vi "Host.vi"() -> ()   [LabVIEW 2025]
uses:
  Controls/panel select 2.ctl
  Controls/home button.ctl
  Controls/manual button 2.ctl
  Controls/edit programs button.ctl
  Controls/diagnostics button.ctl
  Controls/info button 2.ctl
  <vilib>/Handler Framework/CmdQueue/Enqueue Single.vi
  <vilib>/Handler Framework/Handler Framework.lvlib
panel:
  out "Modules":T1
  in  "Page Select":T2
  # "Energized Bake Oven"
  # "Version 1.0.0.0"
  # "RAM Aerospace\nSt. George, UT, 84790\nLabVIEW 2025 Q1\nDQMH-LVOOP-HAL"
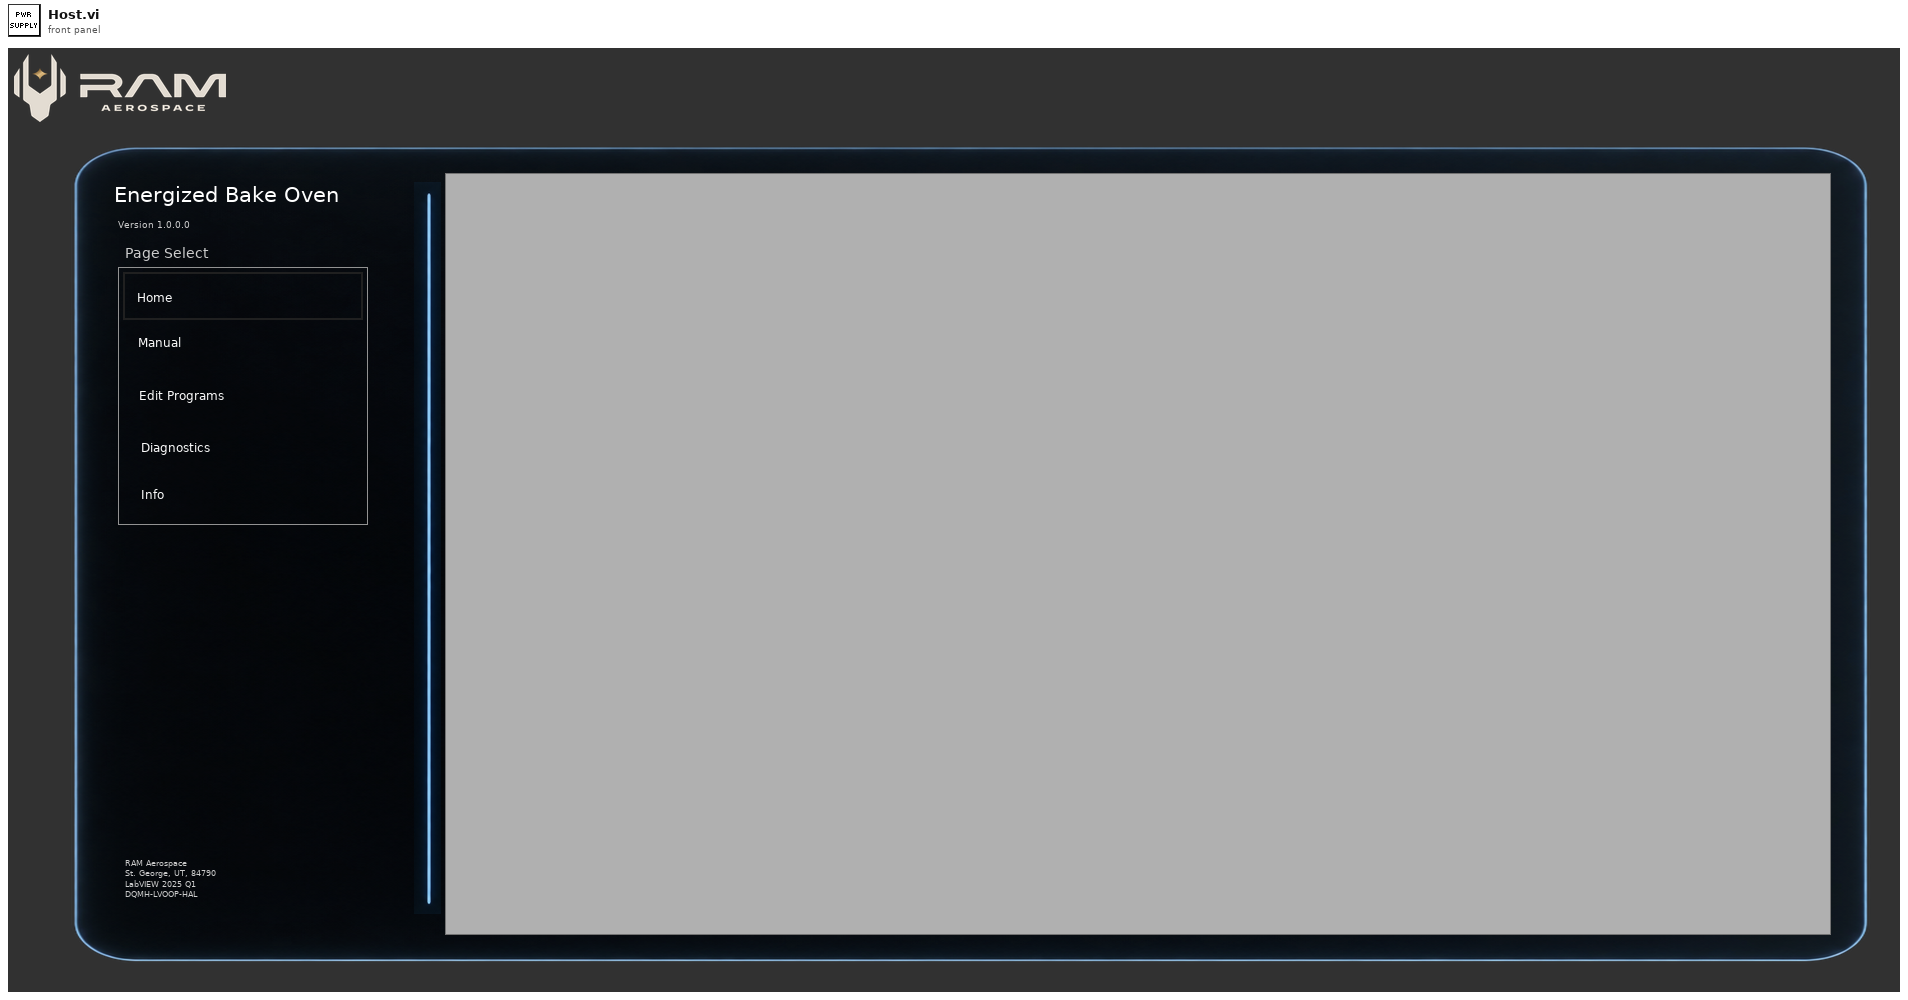
[diagram p1: front panel]
types:
  T1 = cluster{"Module IDs":i32[], "Module Names":string[]}
  T2 = typedef "panel select 2.ctl" = enum32{"Home", "Manual", "Edit Programs", "Diagnostics", "Info"}
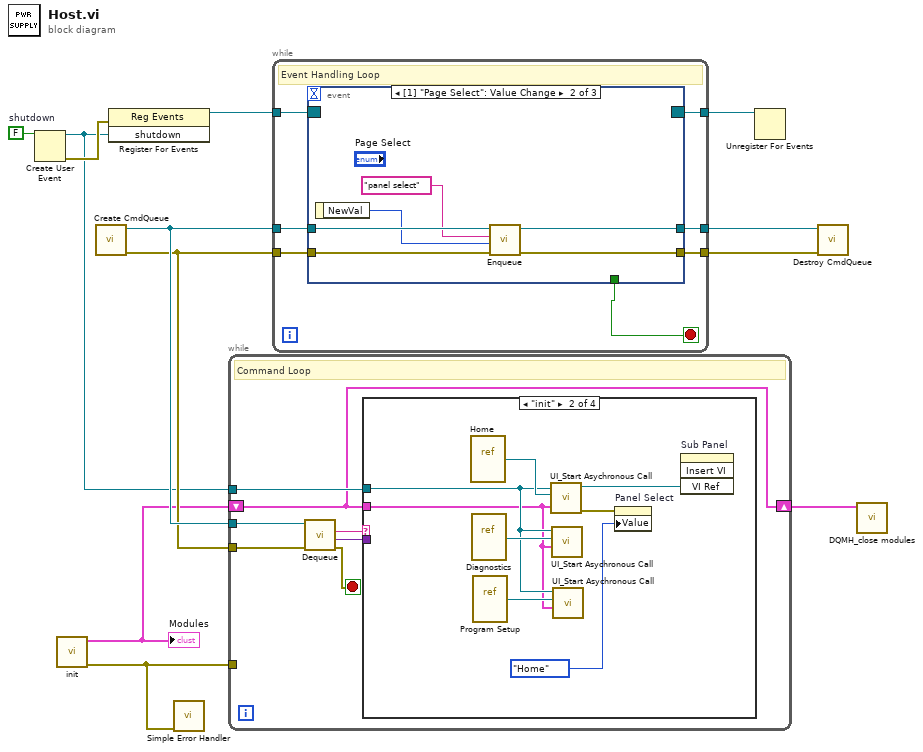
[diagram p0: block diagram]
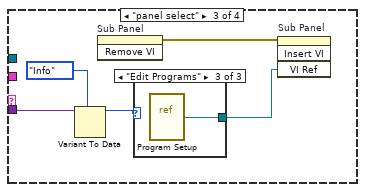
[diagram p3: hidden frame]
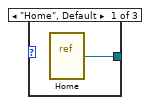
[diagram p4: hidden frame]
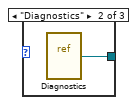
[diagram p5: hidden frame]
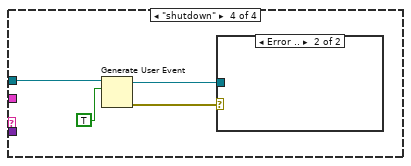
[diagram p6: hidden frame]
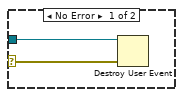
[diagram p7: hidden frame]
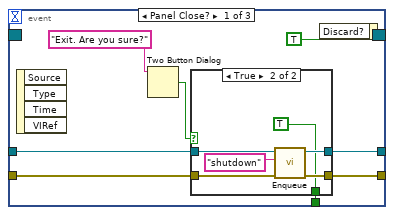
[diagram p8: hidden frame]
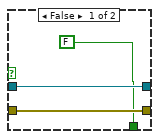
[diagram p9: hidden frame]
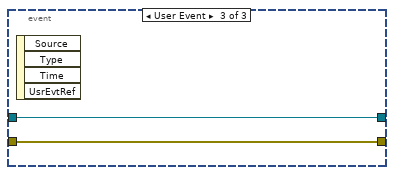
[diagram p10: hidden frame]
diagram:
  w8 = FALSE  # shutdown
  n1 = Create User Event(user event datatype=w8) -> (user event=w4:refnum<user-event>, error out=w5:errorcluster)  [unwired: 1 in]
  n2 = call "init.vi"() -> ("error out"=w1:errorcluster, "Modules"=w3:T1)  [unwired: 10 in]
  "Modules" <- w3
  n3 = call <vilib>:"Create CmdQueue.vi"() -> ("error out"=w9:errorcluster, "CmdQueue out"=w10:refnum<queue>)  [unwired: 10 in]
  n4 = register-events(error in=w5, w4) -> (reference out=w7:refnum<event-registration>)  [unwired: 1 in, 1 out]
  n5 = call <vilib>:"Simple Error Handler.vi"("error in (no error)"=w1) -> ()  [unwired: 4 in, 5 out]
  n6 = while {
    tunnel: w10 -> [w19]
    tunnel: w9 -> [w16]
    tunnel: w4 -> [w15]
    tunnel: w1 -> [_]
    shift-right: [w13] -> w2
    shift-left: w3 -> [w13]
    stop <- w14 stop-if-true
    # "Command Loop"
    n7 = call <vilib>:"Dequeue.vi"("error in (no error)"=w16, "CmdQueue in"=w19) -> ("error out"=w14:errorcluster, "value"=w17:variant, "cmd"=w18:string)  [unwired: 5 in, 2 out]
    n8 = case shown="\"init\"" w18 {
      tunnel: w17 -> [_ _ w32 _]
      tunnel: w15 -> [_ w23 _ w39]
      tunnel: w13 -> [_ w22 _ _]
      frame "False", Default {
      }
      frame "init" {
        n9 = vi-ref "Home.vi"() -> (w27:refnum<vi>)
        n10 = vi-ref "Diagnostics.vi"() -> (w26:refnum<vi>)
        n11 = vi-ref "Program Setup.vi"() -> (w24:refnum<vi>)
        n12 = call "UI_Start Asychronous Call.vi"("DQMH Modules"=w22, "VI Refnum"=w27, "User Event in"=w23) -> ("error out"=w21:errorcluster, "VI ref"=w25:refnum<vi>)  [unwired: 7 in]
        n13 = call "UI_Start Asychronous Call.vi"("DQMH Modules"=w22, "VI Refnum"=w26, "User Event in"=w23) -> ()  [unwired: 7 in, 2 out]
        n14 = call "UI_Start Asychronous Call.vi"("DQMH Modules"=w22, "VI Refnum"=w24, "User Event in"=w23) -> ()  [unwired: 7 in, 2 out]
        n15 = property on="Panel Select" class="RadioBtnsControl (strict)"(error in=w21, "Value"=panel_select_2."Home" ("Panel Select")) -> ()  [unwired: 1 in, 2 out]
        n16 = invoke on="Sub Panel" class="SubPnl" method="Insert VI"("VI Ref"=w25) -> ()  [unwired: 3 in, 4 out]
      }
      frame "panel select" {
        n17 = Variant To Data(type=panel_select_2."Info" ("Panel Select"), Variant=w32) -> (data=w31:T2)  [unwired: 1 in, 1 out]
        n18 = invoke on="Sub Panel" class="SubPnl" method="Remove VI"() -> (error out=w30:errorcluster)  [unwired: 3 in, 2 out]
        n19 = case shown="\"Edit Programs\"" w31 {
          tunnel: [w33 w34 w35] -> w29
          frame "Home", Default {
            n20 = vi-ref "Home.vi"() -> (w33:refnum<vi>)
          }
          frame "Diagnostics" {
            n21 = vi-ref "Diagnostics.vi"() -> (w34:refnum<vi>)
          }
          frame "Edit Programs" {
            n22 = vi-ref "Program Setup.vi"() -> (w35:refnum<vi>)
          }
        }
        n23 = invoke on="Sub Panel" class="SubPnl" method="Insert VI"(error in=w30, "VI Ref"=w29) -> ()  [unwired: 2 in, 4 out]
      }
      frame "shutdown" {
        n24 = Generate User Event(user event=w39, event data cluster=TRUE ("event data")) -> (user event out=w37:refnum<user-event>, error out=w36:errorcluster)  [unwired: 2 in]
        n25 = case shown="Error .." w36 {
          selector: w36 -> [w40 _]
          tunnel: w37 -> [w41 _]
          frame No Error {
            n26 = Destroy User Event(user event=w41, error in=w40) -> ()  [unwired: 1 out]
          }
          frame Error {
          }
        }
      }
    }
  }
  n27 = while {
    tunnel: w10 -> [w46]
    tunnel: [w44] -> w12
    tunnel: w9 -> [w45]
    tunnel: [w43] -> w11
    tunnel: w7 -> [w48]
    tunnel: [w47] -> w6
    stop <- w42 stop-if-true
    # "Event Handling Loop"
    n28 = event shown="[1] \"Page Select\": Value Change" {
      selector: w48 -> [_ _ _]
      dyn-events: [_ _ _] -> w47
      timeout: _ -> [_ _ _]
      tunnel: w46 -> [w56 w71 w73]
      tunnel: w45 -> [w55 w68 w72]
      tunnel: [w53 w70 w73] -> w44
      tunnel: [w52 w69 w72] -> w43
      tunnel: [w49 _ _] -> w42
      event Panel Close? {
        n29 = event-data() -> ()  [unwired: 1 in, 4 out]
        n30 = Two Button Dialog(message="Exit. Are you sure?") -> (T button?=w50:bool)  [unwired: 2 in]
        n31 = case shown="True" w50 {
          tunnel: w56 -> [w59 w64]
          tunnel: w55 -> [w58 w63]
          tunnel: [w59 w62] -> w53
          tunnel: [w58 w61] -> w52
          tunnel: [FALSE ("T button?") TRUE ("T button?")] -> w49
          frame False {
          }
          frame True {
            n32 = call-poly <vilib>:"Enqueue.vi"("error in (no error)"=w63, "Command"="shutdown", "CmdQueue in"=w64) -> ("error out"=w61:errorcluster, "CmdQueue out"=w62:refnum<queue>)  [unwired: 7 in]
          }
        }
        n33 = event-data("Discard?"=TRUE) -> ()  [unwired: 1 in, 1 out]
      }
      event Value Change {
        n34 = event-data() -> ("NewVal"=w66:T2)  [unwired: 1 in]
        n35 = call-poly <vilib>:"Enqueue.vi"("error in (no error)"=w68, "Value"=w66, "Command"="panel select", "CmdQueue in"=w71) -> ("error out"=w69:errorcluster, "CmdQueue out"=w70:refnum<queue>)  [unwired: 6 in]
      }
      event User Event {
        n36 = event-data() -> ()  [unwired: 1 in, 4 out]
      }
    }
  }
  n37 = Unregister For Events(event registration refnum=w6) -> ()  [unwired: 1 in, 1 out]
  n38 = call <vilib>:"Destroy CmdQueue.vi"("error in (no error)"=w11, "CmdQueue in"=w12) -> ()  [unwired: 9 in, 1 out]
  n39 = call "DQMH_close modules.vi"("Modules"=w2) -> ()  [unwired: 11 in]
